vi "Main.vi"() -> ()   [LabVIEW 2019]
uses:
  <vilib>/ProgressBar/Progress Bar Dialog.lvclass
panel:
  in  "Automatic Error Handling":bool
  in  "Contains Compiled Code":bool=TRUE
  in  "Execution:Allow Debugging":bool
  in  "Scan":bool
  in  "Projects":u16(ring) items=["GDevCon 2022.lvproj"]
  # "Performance options\nAll=False"
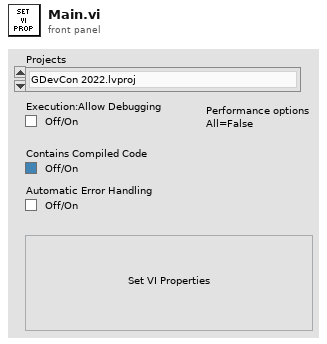
[diagram p1: front panel]
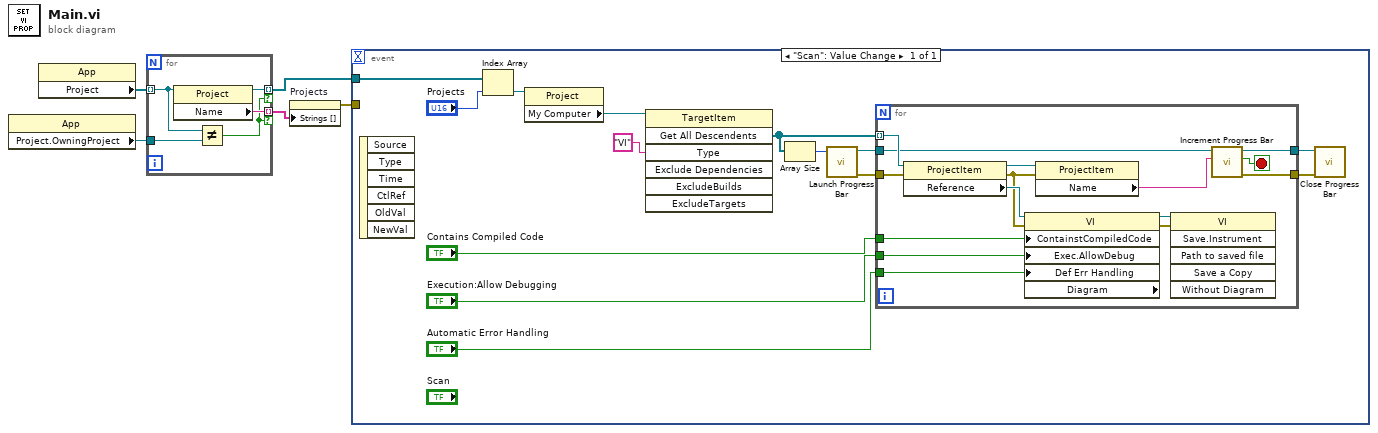
[diagram p0: block diagram]
diagram:
  n1 = property class="App"() -> ("Project.OwningProject"=w2:refnum<vi>)  [unwired: 2 in, 2 out]
  n2 = property class="App"() -> ("Project"=w5:refnum<vi>[])  [unwired: 2 in, 2 out]
  n3 = for {
    tunnel: w5 -> [w8] mode=indexing
    tunnel: [w10] -> w4 mode=indexing if=w6
    tunnel: w2 -> [w9]
    tunnel: [w7] -> w1 mode=indexing if=w6
    n4 = property class="Project"(reference=w8) -> (reference out=w7:refnum<vi>, "Name"=w10:string)  [unwired: 1 in, 1 out]
    n5 = Not Equal?(x=w8, y=w9) -> (x != y?=w6:bool)
  }
  n6 = property on="Projects" class="Ring (strict)"("Strings []"=w4) -> (error out=w3:errorcluster)  [unwired: 2 in, 1 out]
  n7 = event shown="[0] \"Scan\": Value Change" {
    selector: _ -> [_]
    dyn-events: _ -> [_]
    timeout: _ -> [_]
    tunnel: w1 -> [w24]
    tunnel: w3 -> [_]
    event "Scan": Value Change {
      n8 = event-data() -> ()  [unwired: 1 in, 6 out]
      n9 = Index Array(array=w24, index="Projects") -> (element=w22:refnum<vi>)
      n10 = property class="Project"(reference=w22) -> ("My Computer"=w21:refnum<vi>)  [unwired: 1 in, 2 out]
      n11 = invoke class="TargetItem" method="Get All Descendents"(reference=w21, "Type"="VI") -> ("All Descendents"=w14:refnum<vi>[])  [unwired: 5 in, 6 out]
      n12 = Array Size(array=w14) -> (size(s)=w13:i32)
      n13 = call <vilib>:"Launch Progress Bar.vi"("Total Count"=w13) -> ("error out"=w11:errorcluster, "Progress Bar Dialog"=w16:refnum<class "Progress Bar Dialog.lvclass">)  [unwired: 9 in]
      n14 = for {
        tunnel: w14 -> [w39] mode=indexing
        tunnel: "Contains Compiled Code" -> [w36]
        tunnel: "Execution:Allow Debugging" -> [w35]
        tunnel: "Automatic Error Handling" -> [w34]
        tunnel: w16 -> [w32]
        tunnel: [w30] -> w15
        tunnel: [w28] -> w12
        tunnel: w11 -> [w27]
        stop <- w29 stop-if-true
        n15 = property class="ProjectItem"(reference=w39, error in=w27) -> (reference out=w33:refnum<vi>, error out=w25:errorcluster, "Reference"=w37:refnum<vi>)
        n16 = property class="VI" props=["ContainstCompiledCode", "Exec.AllowDebug", "Def Err Handling", "Diagram"](reference=w37, error in=w25, "ContainstCompiledCode"=w36, "Exec.AllowDebug"=w35, "Def Err Handling"=w34) -> (reference out=w38:refnum<vi>, error out=w26:errorcluster)  [unwired: 1 out]
        n17 = property class="ProjectItem"(reference=w33, error in=w25) -> ("Name"=w31:string)  [unwired: 2 out]
        n18 = invoke class="VI" method="Save.Instrument"(reference=w38, error in=w26) -> ()  [unwired: 4 in, 6 out]
        n19 = call <vilib>:"Increment Progress Bar.vi"("Step Name (\"\")"=w31, "Progress Bar Dialog in"=w32) -> ("error out"=w28:errorcluster, "Cancelled?"=w29:bool, "Progress Bar Dialog out"=w30:refnum<class "Progress Bar Dialog.lvclass">)  [unwired: 7 in]
      }
      n20 = call <vilib>:"Close Progress Bar.vi"("error in (no error)"=w12, "Progress Bar Dialog"=w15) -> ()  [unwired: 9 in, 1 out]
    }
  }
